vi "About Robot.vi"(8 "error in (no error)":errorcluster) -> (0 "error out":errorcluster)   [LabVIEW 2017]
panel:
  in  "stop?":bool
  in  "Tab Control":T1(tab)
  # "Autonomous Mapping Robot Platform"
  # "This example demonstrates the software processes and obstacle avoidance algorithm applied to the simulation of an autonomous mapping robot, which can execute multiple missions on command.  This VI explains the simulated components that make up the robot, the connections between components, and the processes that make up the application."
  # "NI Smart Camera"
  # "NI Industrial\nController"
  # "NI CompactRIO"
  # "Digital Position Control and\nbrushless motors"
  # "Laser Range \nFinder (LIDAR)"
  # "Mecanum Wheel"
  # "Mapping and Localization"
  # "Ethernet TCP/IP"
  # "Ethernet\nTCP/IP"
  # "Locomotion and Sensing"
  # "Universal Serial Bus (USB)"
  # "Motion Control Loop"
  # "Brushless\nDC Motor"
  # "Drive"
  # "CAN\nBUS"
  # "Encoder"
  # "Other sensors and \nactuators (touch \nsensor, battery voltage,\ngimbal servos)"
  # "Voltage"
  # "Idle mode"
  # "Teleoperator mode"
  # "Robot Mode\n= Idle"
  # "User control with\njoystick or keyboard"
  # "No operation"
  # "Robot Mode\n= Tele-Op"
  # "Robot Mode\n= Path Following"
  # "Robot Mode\n= Path Following"
  # "Robot Mode\n= Idle"
  # "Robot Mode\n= Tele-Op"
  # "Path Following mode"
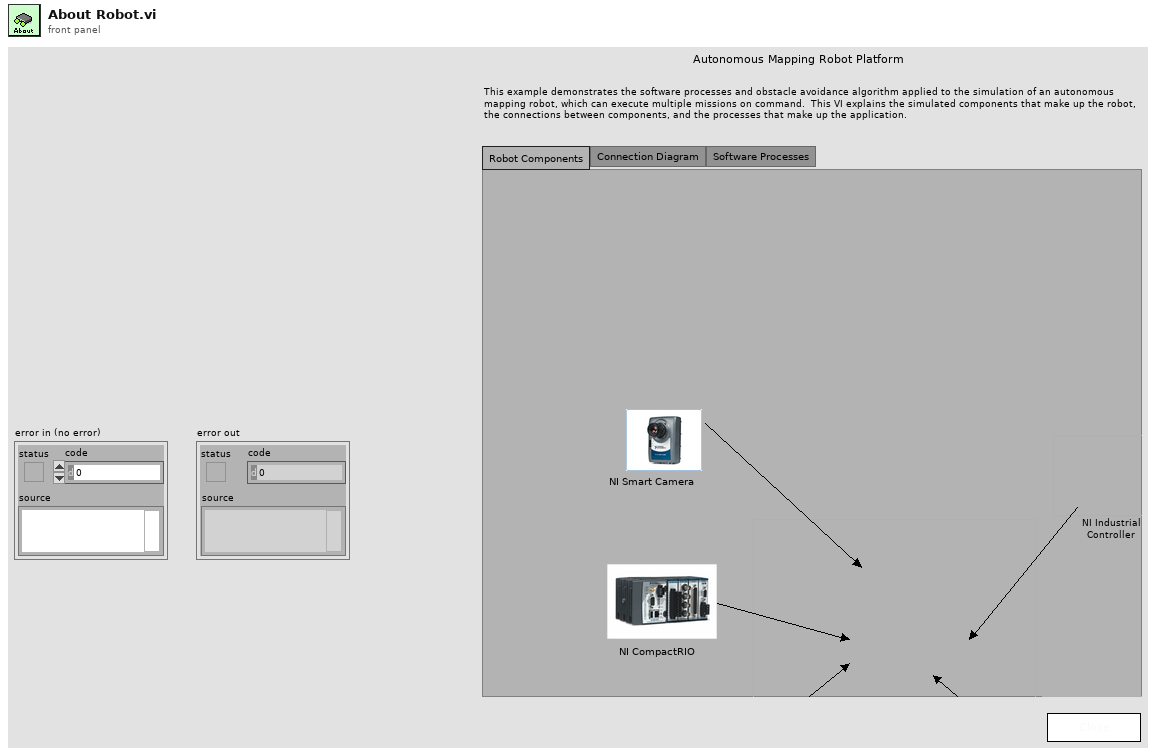
[diagram p1: front panel]
types:
  T1 = enum32{"Robot Components", "Connection Diagram", "Software Processes"}
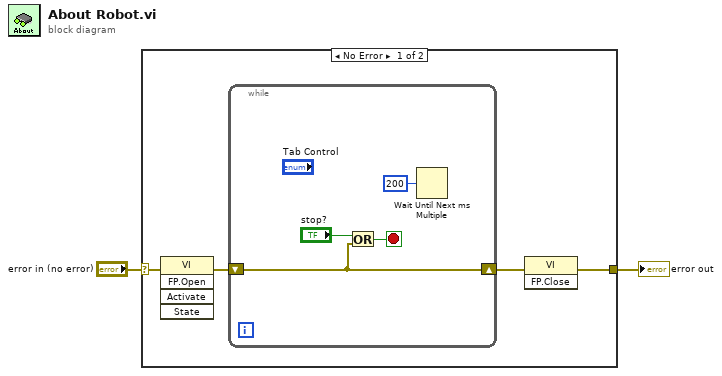
[diagram p0: block diagram]
diagram:
  n1 = case shown="No Error" "error in (no error)" {
    selector: "error in (no error)" -> [w3 w11]
    tunnel: [w4 w11] -> w2
    frame No Error {
      n2 = invoke class="VI" method="FP.Open"(error in=w3) -> (error out=w6:errorcluster)  [unwired: 4 in, 4 out]
      n3 = while {
        shift-right: [w7] -> w5
        shift-left: w6 -> [w7]
        stop <- w10 stop-if-true
        n4 = Or(x="stop?", y=w7) -> (x .or. y?=w10:bool)
        n5 = Wait Until Next ms Multiple(millisecond multiple=u32 200) -> ()  [unwired: 1 out]
      }
      n6 = invoke class="VI" method="FP.Close"(error in=w5) -> (error out=w4:errorcluster)  [unwired: 2 in, 2 out]
    }
    frame Error {
    }
  }
  "error out" <- w2
